vi "PH_PPPA_PowerUnit.ProcState.vi"(0 "i ref in":refnum<vi>, 2 "state timeout":i32=-1, 4 "state":string, 5 "error in (no error)":errorcluster) -> (14 "i ref out":refnum<vi>, 18 "next state":string, 19 "error out":errorcluster)   [LabVIEW 2014, in "PH_PPPA_PowerUnit.lvlib"]
doc: "This VI represents part of the internal state machine of the object. All methods that are needed to implement the required functionality of the state machine will be called from THIS VI. Add your code here."
uses:
  PH_PPPA_PowerUnit.lvlib
  PH_Basics/PH_PowerUnit_BaseClass/PH_PowerUnit_BaseClass.SM States.ctl
  CS_Core/CSSystem/CoreDefs/CoreDefs.error_type.ctl
  CS_Core/CSSystem/CoreLib/CoreLib.lvlib
  CS_Core/BaseSM/BaseSM.lvlib
  PH_Basics/PH_PSDBWriter/PH_PSDBWriter.lvlib
  PH_Devices/PH_Beckhoff_PP_PU/PH_Beckhoff_PP_PU.lvlib
  PH_Basics/PH_PowerUnit_BaseClass/PH_PowerUnit_BaseClass.lvlib
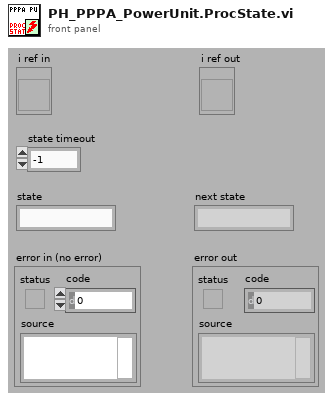
[diagram p1: front panel]
types:
  T1 = typedef "PH_PowerUnit_BaseClass.lvlib/PH_PowerUnit_BaseClass.SM States.ctl" = enum16{".", "Stand by", "Switch PU on", "Configure", "Set Default Voltage", "Set STANDBY", "Set READY", "Wait for Shot Cmd", "Open Dump Rods", "Open Ross Relais", "Close Ross Relais", "Switch PSU on", "Switch PSU off", "Charge", "Switch GD Channel on", "Close Dump Rods", "Rods-TO", "RR-TO", "PSU-TO", "Trigger-TO"}
  T2 = typedef "CoreDefs.error_type.ctl" = enum16{"no error", "can't load process", "can't unload process", "process does not exist", "can't install process", "can't remove process", "unknown function", "time out", "can't execute function", "duplicate queue name", "super not found", "caller queue invalid", "can't ping process", "unknown error", "VISA Error", "VISA timeout", "GPIB timeout", "GPIB error", "communication error", "data type mismatch", "can't read data from OPC server", "can't write data to OPC server", "OET error", "function not implemented", "process already exists", "invalid Shared Variable name", "error writing Shared Variable", "error reading Shared Variable", "invalid client name", "corrupt database", "unknown class", "call not authorized", "parameter out of range", "OET timeout: can't get data to modify", "invalid queue name", "requested operation incompatible with current state", "event undefined", "event disabled", "state undefined", "caller is not a friend", "EventBuilder: bad eventID", "EventBuilder: no DAQ devices", "a thread must not stop itself", "UNUSED ELEMENT4", "DiscArchiver: eventData incomplete", "DiscArchiver: eventData does not belong to run", "DiscArchiver: can't open file", "DiscArchiver: can't write to file", "DiscArchiver: available disc space low", "can't acquire semaphore", "error reading data from database", "notifier object is not existing", "can't register process", "can't unregister process", "illegal event type", "object disabled", "object already exists", "can't change state", "Instrument not found", "no connection to remote node", "invalid reference", "N/A", "UNUSED ELEMENT 1", "element not found", "illegal TCP/IP connection detected", "object does not exist", "invalid access ID", "unknown CS system", "invalid privilige", "unsupported data type", "unsupported server type", "IO server already exists", "Shared Variable already exists"}
  T3 = typedef "PH_PowerUnit_BaseClass.lvlib/PH_PowerUnit_BaseClass.i attribute.ctl" = cluster{"Constructor finished":bool, "PU":cluster{"In use":bool, "Service ID in use":i32, "GUI Ref":refnum<vi>}, "Enabling":cluster{"State":T4, "GUI Ref":refnum<vi>}, "Timing":cluster{"Last Shot":dbl, "Time between Shots [Sec]":dbl, "Waiting Time over?":bool, "Service ID Waiting Time":i32, "GUI Ref":refnum<vi>, "Instance":cluster{"Status":T5, "linked?":bool, "GUI Ref":refnum<vi>}}, "Sequencer":cluster{"SM State":string, "GUI Ref":refnum<vi>, "linked":bool}, "Subscribed Trendmssgs":cluster{"Tagname":string, "Status":T5, "linked?":bool, "Shot Condition":T5, "GUI Ref":refnum<vi>}[], "PP PU":T6, "Default Voltage (V)":dbl, "GUI Refs":T7, "PSDB data":cluster{"Shot Voltage [V]":dbl, "State TO SM":T1, "Write 2 early":bool}, "State TO SM":T1}
  T4 = typedef "PH_SystemInformation.lvlib/PH_SystemInformationEnabling State.ctl" = i32
  T5 = typedef "PH_StatusHandler.lvlib/PH_StatusHandler.Status.ctl" = i16
  T6 = typedef "PH_PP_Common.lvlib/PH_PP_Common.PUs.ctl" = enum16{"no Info", "PA-19mm-1", "PA-19mm-2", "PA-45mm-PILC", "PA-45mm-MAIN", "MA-PU-1", "MA-PU-2", "MA-PU-3", "MA-PU-4", "MA-PU-5", "MA-PU-6", "MA-FR", "MA-PILC", "PA-45mm-DP"}
  T7 = typedef "PH_PowerUnit_BaseClass.lvlib/PH_PowerUnit_BaseClass.GUI Refs.ctl" = cluster{"Delete Inst":refnum<vi>, "State TO SM":refnum<vi>, "State SM":refnum<vi>, "Fire":refnum<vi>}
  T8 = typedef "PH_PPPA_PowerUnit.lvlib/PH_PPPA_PowerUnit.i attribute.ctl" = cluster{"GUI Refs":cluster{"Ignitron":refnum<vi>, "Rossrelais":refnum<vi>, "Set Voltage":refnum<vi>, "PSU":refnum<vi>, "EOC":refnum<vi>, "Trigger":refnum<vi>}, "Ignitron":T9, "PSU":T10, "Dump Ross Relais":T11, "Trigger":cluster{"State Device":T5, "linked?":bool}, "Timing Settings":cluster{"Prdc Fast?":bool, "Default Value Periodic Interval":i32, "Mercury on since":dbl, "Warm up Time Mercury [s]":dbl}, "Set Voltage [V]":dbl, "19er Ignitionbox":string}
  T9 = typedef "PH_PP_Common.lvlib/PH_PP_Common.Ignitron Attributes.ctl" = cluster{"State Device":T5, "linked?":bool}
  T10 = typedef "PH_PP_Common.lvlib/PH_PP_Common.PSU Attributes.ctl" = cluster{"lower limit [V]":dbl, "upper limit [V]":dbl, "Voltage set":bool, "State Device":T5, "linked?":bool}
  T11 = typedef "PH_PP_Common.lvlib/PH_PP_Common.Ross Relais Attributes.ctl" = cluster{"State Device":T5, "linked?":bool}
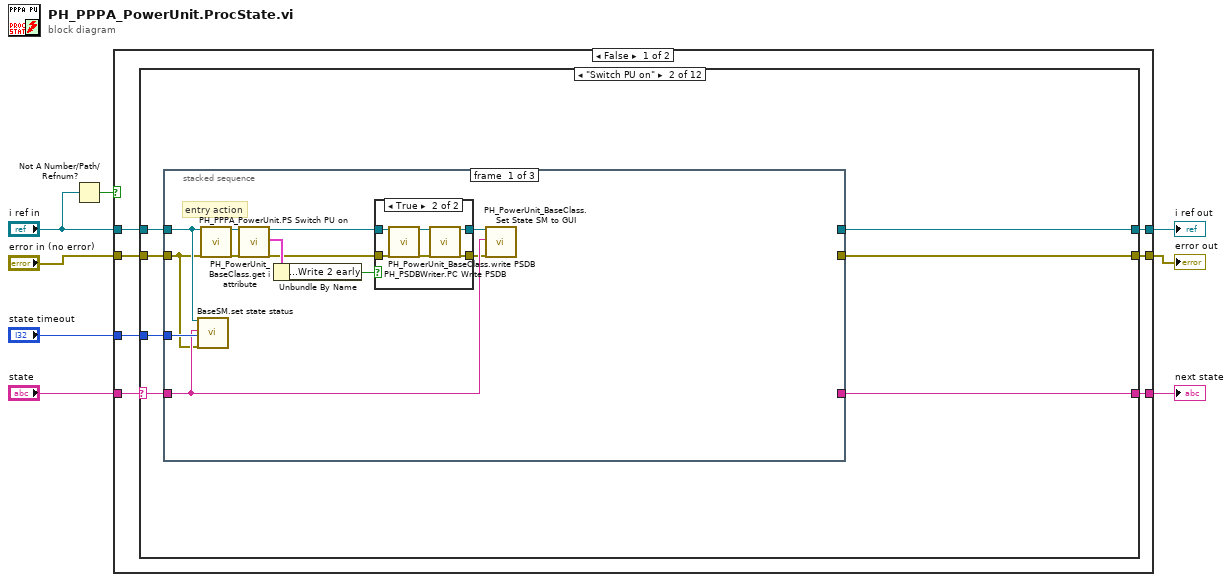
[diagram p0: block diagram]
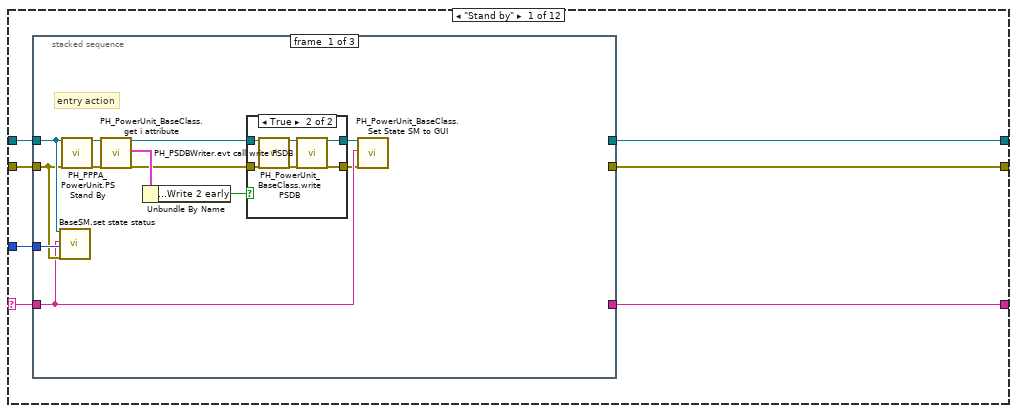
[diagram p2: hidden frame]
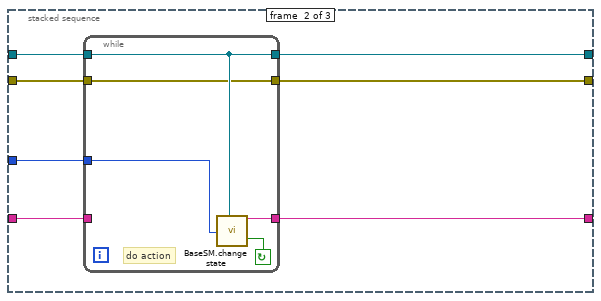
[diagram p4: hidden frame]
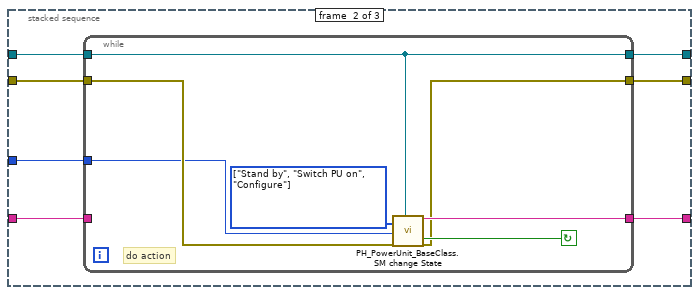
[diagram p7: hidden frame]
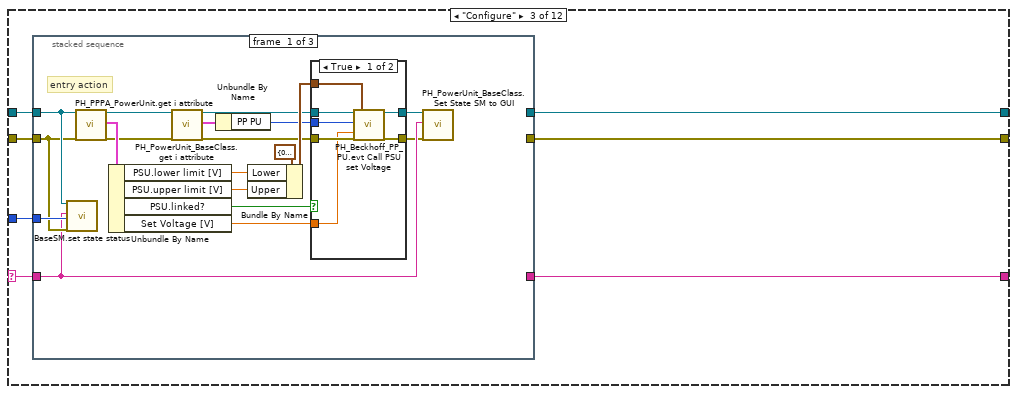
[diagram p9: hidden frame]
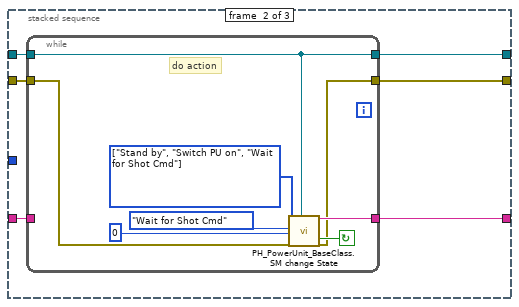
[diagram p11: hidden frame]
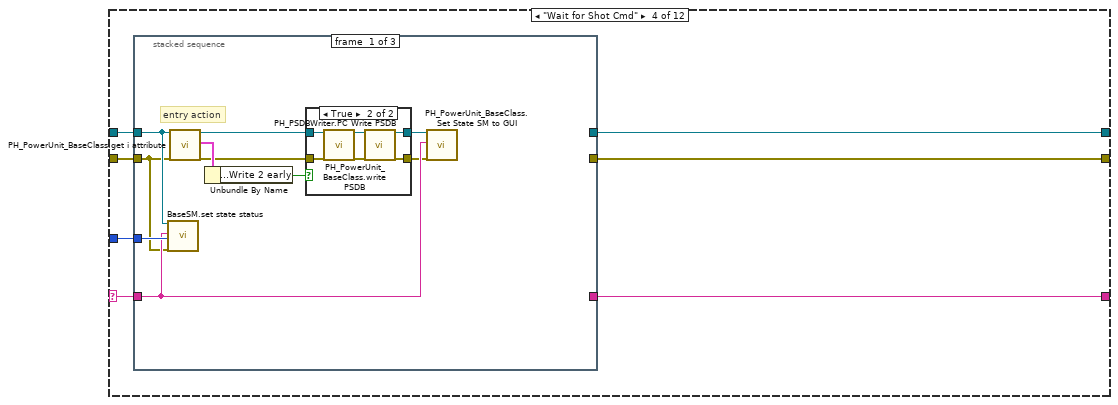
[diagram p13: hidden frame]
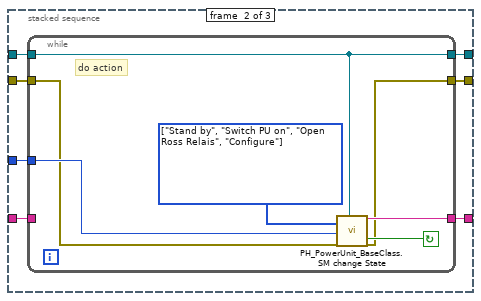
[diagram p15: hidden frame]
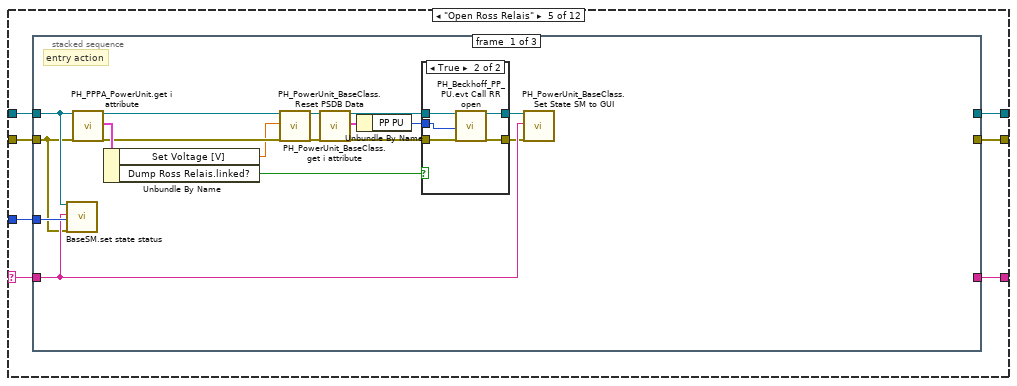
[diagram p17: hidden frame]
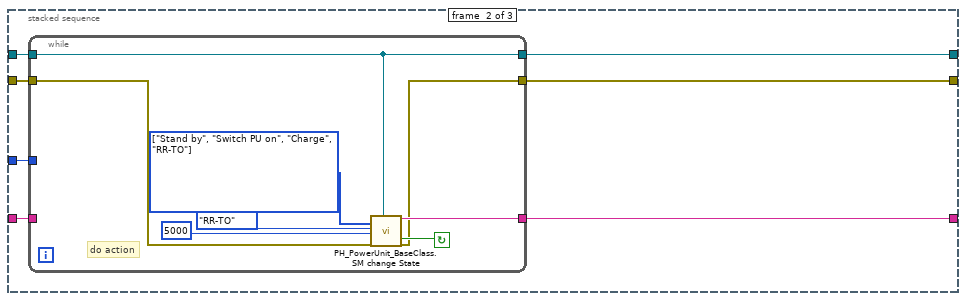
[diagram p19: hidden frame]
diagram:
  n1 = Not A Number/Path/Refnum?(number/path/refnum="i ref in") -> (NaN/Path/Refnum?=w2:bool)
  n2 = case shown="False" w2 {
    tunnel: "i ref in" -> [w15 w435]
    tunnel: [w14 w435] -> w8
    tunnel: "state" -> [w13 w432]
    tunnel: [w12 w432] -> w6
    tunnel: "state timeout" -> [w11 _]
    tunnel: "error in (no error)" -> [w10 _]
    tunnel: [w9 w433] -> w3
    frame False {
      n3 = case shown="\"Switch PU on\"" w13 {
        selector: w13 -> [w22 w61 w102 w151 w190 w236 w298 w323 w350 w377 w404 w426]
        tunnel: w15 -> [w20 w59 w100 w149 w188 w234 w296 w321 w348 w375 w402 w431]
        tunnel: [w19 w58 w99 w148 w187 w233 w295 w320 w347 w374 w401 w430] -> w14
        tunnel: [w21 w60 w101 w150 w189 w235 w297 w322 w349 w376 w403 w425] -> w12
        tunnel: w11 -> [w18 w57 w98 w147 w186 w232 w294 w319 w346 w373 w400 w427]
        tunnel: w10 -> [w17 w56 w97 w146 w185 w231 w293 w318 w345 w372 w399 w429]
        tunnel: [w16 w55 w96 w145 w184 w230 w292 w317 w344 w371 w398 w428] -> w9
        frame "Stand by" {
          n4 = stacked-sequence {
            tunnel: w22 -> [w31 w49 _]
            tunnel: [_ w48 _] -> w21
            tunnel: w20 -> [w33 w46 _]
            tunnel: [_ w45 _] -> w19
            tunnel: w18 -> [w34 w47 _]
            tunnel: w17 -> [w32 w43 _]
            tunnel: [_ w44 _] -> w16
            frame #0 {
              # "entry action"
              n5 = call "BaseSM.set state status.vi"("i ref in"=w33, "stateStatus"=w31, "ms timeout (10000)"=w34, "error in (no error)"=w32) -> ()  [unwired: 13 in, 3 out]
              n6 = call "PH_PPPA_PowerUnit.PS Stand By.vi"("i ref in"=w33, "error in (no error)"=w32) -> ("i ref out"=w29:refnum<vi>, "error out"=w28:errorcluster)  [unwired: 16 in]
              n7 = call "PH_PowerUnit_BaseClass.get i attribute.vi"("i ref in"=w29, "error in (no error)"=w28) -> ("i ref out"=w27:refnum<vi>, "i attribute"=w30:T3, "error out"=w26:errorcluster)  [unwired: 15 in]
              n8 = Unbundle By Name(w30) -> ("PSDB data.Write 2 early"=w25:bool)
              n9 = case shown="True" w25 {
                tunnel: [w36 w38] -> w24
                tunnel: [w35 w37] -> w23
                tunnel: w27 -> [w36 w42]
                tunnel: w26 -> [w35 w41]
                frame False {
                }
                frame True {
                  n10 = call "PH_PowerUnit_BaseClass.write PSDB.vi"("i ref in"=w42, "error IO"=w41) -> ("i ref out"=w39:refnum<vi>, "error out"=w40:errorcluster)  [unwired: 16 in]
                  n11 = call "PH_PSDBWriter.evt call write PSDB.vi"("i ref in"=w39, "error in (no error)"=w40) -> ("i ref out"=w38:refnum<vi>, "error out"=w37:errorcluster)  [unwired: 16 in]
                }
              }
              n12 = call "PH_PowerUnit_BaseClass.Set State SM to GUI.vi"("i ref in"=w24, "State SM"=w31, "error in (no error)"=w23) -> ()  [unwired: 15 in, 2 out]
            }
            frame #1 {
              n13 = while {
                tunnel: w47 -> [w52]
                tunnel: [w54] -> w48
                tunnel: w49 -> [_]
                tunnel: w46 -> [w51]
                tunnel: [w51] -> w45
                tunnel: [w50] -> w44
                tunnel: w43 -> [w50]
                stop <- w53 continue-if-true
                # "do action"
                n14 = call "BaseSM.change state.vi"("wait time [ms]"=w52, "i ref in"=w51) -> ("next state"=w54:string, "continue loop"=w53:bool)  [unwired: 14 in, 2 out]
              }
            }
            frame #2 {
              # "exit action"
            }
          }
        }
        frame "Switch PU on" {
          n15 = stacked-sequence {
            tunnel: w61 -> [w72 w88 _]
            tunnel: [_ w87 _] -> w60
            tunnel: w59 -> [w71 w86 _]
            tunnel: [_ w85 _] -> w58
            tunnel: w57 -> [w73 w82 _]
            tunnel: w56 -> [w70 w83 _]
            tunnel: [_ w84 _] -> w55
            frame #0 {
              # "entry action"
              n16 = call "BaseSM.set state status.vi"("i ref in"=w71, "stateStatus"=w72, "ms timeout (10000)"=w73, "error in (no error)"=w70) -> ()  [unwired: 13 in, 3 out]
              n17 = call "PH_PPPA_PowerUnit.PS Switch PU on.vi"("i ref in"=w71, "error in (no error)"=w70) -> ("i ref out"=w65:refnum<vi>, "error out"=w64:errorcluster)  [unwired: 16 in]
              n18 = call "PH_PowerUnit_BaseClass.get i attribute.vi"("i ref in"=w65, "error in (no error)"=w64) -> ("i ref out"=w68:refnum<vi>, "i attribute"=w69:T3, "error out"=w67:errorcluster)  [unwired: 15 in]
              n19 = Unbundle By Name(w69) -> ("PSDB data.Write 2 early"=w66:bool)
              n20 = case shown="True" w66 {
                tunnel: w68 -> [w75 w77]
                tunnel: w67 -> [w74 w76]
                tunnel: [w75 w79] -> w63
                tunnel: [w74 w78] -> w62
                frame False {
                }
                frame True {
                  n21 = call "PH_PowerUnit_BaseClass.write PSDB.vi"("i ref in"=w77, "error IO"=w76) -> ("i ref out"=w80:refnum<vi>, "error out"=w81:errorcluster)  [unwired: 16 in]
                  n22 = call "PH_PSDBWriter.PC Write PSDB.vi"("i ref in"=w80, "error IO"=w81) -> ("i ref out"=w79:refnum<vi>, "error out"=w78:errorcluster)  [unwired: 16 in]
                }
              }
              n23 = call "PH_PowerUnit_BaseClass.Set State SM to GUI.vi"("i ref in"=w63, "State SM"=w72, "error in (no error)"=w62) -> ()  [unwired: 15 in, 2 out]
            }
            frame #1 {
              n24 = while {
                tunnel: [w95] -> w87
                tunnel: w88 -> [_]
                tunnel: w86 -> [w93]
                tunnel: [w93] -> w85
                tunnel: [w91] -> w84
                tunnel: w83 -> [w92]
                tunnel: w82 -> [w90]
                stop <- w94 continue-if-true
                w89 = T1[] [enum."Stand by", enum."Switch PU on", enum."Configure"] items=[".", "Stand by", "Switch PU on", "Configure", "Set Default Voltage", "Set STANDBY", "Set READY", "Wait for Shot Cmd", "Open Dump Rods", "Open Ross Relais", "Close Ross Relais", "Switch PSU on", "Switch PSU off", "Charge", "Switch GD Channel on", "Close Dump Rods", "Rods-TO", "RR-TO", "PSU-TO", "Trigger-TO"] ("allowed next states")
                # "do action"
                n25 = call "PH_PowerUnit_BaseClass.SM change State.vi"("allowed next states"=w89, "wait time [ms]"=w90, "error in (no error)"=w92, "VI in"=w93) -> ("next state"=w95:string, "continue loop"=w94:bool, "error out"=w91:errorcluster)  [unwired: 13 in]
              }
            }
            frame #2 {
              # "exit action"
            }
          }
        }
        frame "Configure" {
          n26 = stacked-sequence {
            tunnel: w102 -> [w118 w136 _]
            tunnel: [_ w135 _] -> w101
            tunnel: w100 -> [w120 w134 _]
            tunnel: [_ w133 _] -> w99
            tunnel: w98 -> [w121 _ _]
            tunnel: w97 -> [w119 w131 _]
            tunnel: [_ w132 _] -> w96
            frame #0 {
              # "entry action"
              n27 = call "BaseSM.set state status.vi"("i ref in"=w120, "stateStatus"=w118, "ms timeout (10000)"=w121, "error in (no error)"=w119) -> ()  [unwired: 13 in, 3 out]
              n28 = call "PH_PPPA_PowerUnit.get i attribute.vi"("i ref in"=w120, "error in (no error)"=w119) -> ("i ref out"=w106:refnum<vi>, "i attribute"=w117:T8, "error out"=w105:errorcluster)  [unwired: 15 in]
              n29 = Unbundle By Name(w117) -> ("PSU.lower limit [V]"=w112:dbl, "PSU.upper limit [V]"=w111:dbl, "PSU.linked?"=w115:bool, "Set Voltage [V]"=w116:dbl)
              n30 = call "PH_PowerUnit_BaseClass.get i attribute.vi"("i ref in"=w106, "error in (no error)"=w105) -> ("i ref out"=w109:refnum<vi>, "i attribute"=w108:T3, "error out"=w110:errorcluster)  [unwired: 15 in]
              n31 = Unbundle By Name(w108) -> ("PP PU"=w107:T6)
              n32 = Bundle By Name(cluster=cluster{"Lower":dbl, "Upper":dbl} {"Lower"=0.0, "Upper"=0.0} ("Limits [V]"), "Lower"=w112, "Upper"=w111) -> (w113:cluster{"Lower":dbl, "Upper":dbl})
              n33 = case shown="True" w115 {
                tunnel: w109 -> [w128 w130]
                tunnel: w110 -> [w127 w129]
                tunnel: w116 -> [w126 _]
                tunnel: [w125 w130] -> w104
                tunnel: [w124 w129] -> w103
                tunnel: w113 -> [w123 _]
                tunnel: w107 -> [w122 _]
                frame True {
                  n34 = call "PH_Beckhoff_PP_PU.evt Call PSU set Voltage.vi"("i ref in"=w128, "PU"=w122, "Voltage to set [V]"=w126, "error in"=w127, "Limits [V]"=w123) -> ("i ref out"=w125:refnum<vi>, "error out"=w124:errorcluster)  [unwired: 13 in]
                }
                frame False {
                }
              }
              n35 = call "PH_PowerUnit_BaseClass.Set State SM to GUI.vi"("i ref in"=w104, "State SM"=w118, "error in (no error)"=w103) -> ()  [unwired: 15 in, 2 out]
            }
            frame #1 {
              n36 = while {
                tunnel: [w144] -> w135
                tunnel: w136 -> [_]
                tunnel: w134 -> [w142]
                tunnel: [w142] -> w133
                tunnel: [w140] -> w132
                tunnel: w131 -> [w141]
                stop <- w143 continue-if-true
                w137 = T1[] [enum."Stand by", enum."Switch PU on", enum."Wait for Shot Cmd"] items=[".", "Stand by", "Switch PU on", "Configure", "Set Default Voltage", "Set STANDBY", "Set READY", "Wait for Shot Cmd", "Open Dump Rods", "Open Ross Relais", "Close Ross Relais", "Switch PSU on", "Switch PSU off", "Charge", "Switch GD Channel on", "Close Dump Rods", "Rods-TO", "RR-TO", "PSU-TO", "Trigger-TO"] ("allowed next states")
                # "do action"
                n37 = call "PH_PowerUnit_BaseClass.SM change State.vi"("allowed next states"=w137, "default state"=PH_PowerUnit_BaseClass.SM_States."Wait for Shot Cmd", "wait time [ms]"=0 ("wait time"), "error in (no error)"=w141, "VI in"=w142) -> ("next state"=w144:string, "continue loop"=w143:bool, "error out"=w140:errorcluster)  [unwired: 12 in]
              }
            }
            frame #2 {
              # "exit action"
            }
          }
        }
        frame "Wait for Shot Cmd" {
          n38 = stacked-sequence {
            tunnel: w151 -> [w160 w176 _]
            tunnel: [_ w175 _] -> w150
            tunnel: w149 -> [w155 w173 _]
            tunnel: [_ w172 _] -> w148
            tunnel: w147 -> [w161 w174 _]
            tunnel: w146 -> [w154 w170 _]
            tunnel: [_ w171 _] -> w145
            frame #0 {
              # "entry action"
              n39 = call "BaseSM.set state status.vi"("i ref in"=w155, "stateStatus"=w160, "ms timeout (10000)"=w161, "error in (no error)"=w154) -> ()  [unwired: 13 in, 3 out]
              n40 = call "PH_PowerUnit_BaseClass.get i attribute.vi"("i ref in"=w155, "error in (no error)"=w154) -> ("i ref out"=w158:refnum<vi>, "i attribute"=w159:T3, "error out"=w157:errorcluster)  [unwired: 15 in]
              n41 = Unbundle By Name(w159) -> ("PSDB data.Write 2 early"=w156:bool)
              n42 = case shown="True" w156 {
                tunnel: w158 -> [w163 w165]
                tunnel: w157 -> [w162 w164]
                tunnel: [w163 w167] -> w153
                tunnel: [w162 w166] -> w152
                frame False {
                }
                frame True {
                  n43 = call "PH_PowerUnit_BaseClass.write PSDB.vi"("i ref in"=w165, "error IO"=w164) -> ("i ref out"=w168:refnum<vi>, "error out"=w169:errorcluster)  [unwired: 16 in]
                  n44 = call "PH_PSDBWriter.PC Write PSDB.vi"("i ref in"=w168, "error IO"=w169) -> ("i ref out"=w167:refnum<vi>, "error out"=w166:errorcluster)  [unwired: 16 in]
                }
              }
              n45 = call "PH_PowerUnit_BaseClass.Set State SM to GUI.vi"("i ref in"=w153, "State SM"=w160, "error in (no error)"=w152) -> ()  [unwired: 15 in, 2 out]
            }
            frame #1 {
              n46 = while {
                tunnel: w174 -> [w181]
                tunnel: [w183] -> w175
                tunnel: w176 -> [_]
                tunnel: w173 -> [w180]
                tunnel: [w180] -> w172
                tunnel: [w178] -> w171
                tunnel: w170 -> [w179]
                stop <- w182 continue-if-true
                w177 = T1[] [enum."Stand by", enum."Switch PU on", enum."Open Ross Relais", enum."Configure"] items=[".", "Stand by", "Switch PU on", "Configure", "Set Default Voltage", "Set STANDBY", "Set READY", "Wait for Shot Cmd", "Open Dump Rods", "Open Ross Relais", "Close Ross Relais", "Switch PSU on", "Switch PSU off", "Charge", "Switch GD Channel on", "Close Dump Rods", "Rods-TO", "RR-TO", "PSU-TO", "Trigger-TO"] ("allowed next states")
                # "do action"
                n47 = call "PH_PowerUnit_BaseClass.SM change State.vi"("allowed next states"=w177, "wait time [ms]"=w181, "error in (no error)"=w179, "VI in"=w180) -> ("next state"=w183:string, "continue loop"=w182:bool, "error out"=w178:errorcluster)  [unwired: 13 in]
              }
            }
            frame #2 {
              # "exit action"
            }
          }
        }
        frame "Open Ross Relais" {
          n48 = stacked-sequence {
            tunnel: w190 -> [w205 w221 _]
            tunnel: [_ w220 _] -> w189
            tunnel: w188 -> [w199 w218 _]
            tunnel: [_ w217 _] -> w187
            tunnel: w186 -> [w207 w219 _]
            tunnel: w185 -> [w198 w215 _]
            tunnel: [_ w216 _] -> w184
            frame #0 {
              # "entry action"
              n49 = call "BaseSM.set state status.vi"("i ref in"=w199, "stateStatus"=w205, "ms timeout (10000)"=w207, "error in (no error)"=w198) -> ()  [unwired: 13 in, 3 out]
              n50 = call "PH_PPPA_PowerUnit.get i attribute.vi"("i ref in"=w199, "error in (no error)"=w198) -> ("i ref out"=w195:refnum<vi>, "i attribute"=w206:T8, "error out"=w197:errorcluster)  [unwired: 15 in]
              n51 = Unbundle By Name(w206) -> ("Set Voltage [V]"=w193:dbl, "Dump Ross Relais.linked?"=w204:bool)
              n52 = call "PH_PowerUnit_BaseClass.Reset PSDB Data.vi"("VI in"=w195, "PSDB data.Shot Voltage [V]"=w193, "error in (no error)"=w197) -> ("VI out"=w194:refnum<vi>, "error out"=w196:errorcluster)  [unwired: 15 in]
              n53 = call "PH_PowerUnit_BaseClass.get i attribute.vi"("i ref in"=w194, "error in (no error)"=w196) -> ("i ref out"=w202:refnum<vi>, "i attribute"=w201:T3, "error out"=w203:errorcluster)  [unwired: 15 in]
              n54 = Unbundle By Name(w201) -> ("PP PU"=w200:T6)
              n55 = case shown="True" w204 {
                tunnel: w202 -> [w209 w214]
                tunnel: w203 -> [w208 w213]
                tunnel: [w208 w212] -> w191
                tunnel: [w209 w211] -> w192
                tunnel: w200 -> [_ w210]
                frame False {
                }
                frame True {
                  n56 = call "PH_Beckhoff_PP_PU.evt Call RR open.vi"("i ref in"=w214, "PU"=w210, "error in"=w213) -> ("i ref out"=w211:refnum<vi>, "error out"=w212:errorcluster)  [unwired: 15 in]
                }
              }
              n57 = call "PH_PowerUnit_BaseClass.Set State SM to GUI.vi"("i ref in"=w192, "State SM"=w205, "error in (no error)"=w191) -> ()  [unwired: 15 in, 2 out]
            }
            frame #1 {
              n58 = while {
                tunnel: w219 -> [_]
                tunnel: [w229] -> w220
                tunnel: w221 -> [_]
                tunnel: w218 -> [w227]
                tunnel: [w227] -> w217
                tunnel: [w224] -> w216
                tunnel: w215 -> [w225]
                stop <- w228 continue-if-true
                w222 = T1[] [enum."Stand by", enum."Switch PU on", enum."Charge", enum."RR-TO"] items=[".", "Stand by", "Switch PU on", "Configure", "Set Default Voltage", "Set STANDBY", "Set READY", "Wait for Shot Cmd", "Open Dump Rods", "Open Ross Relais", "Close Ross Relais", "Switch PSU on", "Switch PSU off", "Charge", "Switch GD Channel on", "Close Dump Rods", "Rods-TO", "RR-TO", "PSU-TO", "Trigger-TO"] ("allowed next states")
                # "do action"
                n59 = call "PH_PowerUnit_BaseClass.SM change State.vi"("allowed next states"=w222, "default state"=PH_PowerUnit_BaseClass.SM_States."RR-TO", "wait time [ms]"=5000 ("wait time"), "error in (no error)"=w225, "VI in"=w227) -> ("next state"=w229:string, "continue loop"=w228:bool, "error out"=w224:errorcluster)  [unwired: 12 in]
              }
            }
            frame #2 {
              # "exit action"
            }
          }
        }
        frame "Charge" {
          n60 = stacked-sequence {
            tunnel: w236 -> [w244 w283 _]
            tunnel: [_ w282 _] -> w235
            tunnel: w234 -> [w249 w281 _]
            tunnel: [_ w280 _] -> w233
            tunnel: w232 -> [w250 _ _]
            tunnel: w231 -> [w248 w278 _]
            tunnel: [_ w279 _] -> w230
            frame #0 {
              # "entry action"
              n61 = call "BaseSM.set state status.vi"("i ref in"=w249, "stateStatus"=w244, "ms timeout (10000)"=w250, "error in (no error)"=w248) -> ()  [unwired: 13 in, 3 out]
              n62 = call "PH_PPPA_PowerUnit.get i attribute.vi"("i ref in"=w249, "error in (no error)"=w248) -> ("i ref out"=w237:refnum<vi>, "i attribute"=w247:T8, "error out"=w238:errorcluster)  [unwired: 15 in]
              n63 = Unbundle By Name(w247) -> ("PSU.linked?"=w243:bool)
              n64 = call "PH_PowerUnit_BaseClass.get i attribute.vi"("i ref in"=w237, "error in (no error)"=w238) -> ("i ref out"=w241:refnum<vi>, "i attribute"=w240:T3, "error out"=w242:errorcluster)  [unwired: 15 in]
              n65 = Unbundle By Name(w240) -> ("PP PU"=w239:T6)
              n66 = case shown="True" w243 {
                tunnel: w241 -> [w261 w277]
                tunnel: w242 -> [w260 w276]
                tunnel: [w252 w276] -> w245
                tunnel: [w251 w277] -> w246
                tunnel: w239 -> [w259 _]
                frame True {
                  n67 = flat-sequence {
                    tunnel: w261 -> [w266]
                    tunnel: w260 -> [w264]
                    tunnel: w259 -> [w262]
                    tunnel: [w265] -> w258
                    tunnel: [w263] -> w257
                    tunnel: [w262] -> w256
                    tunnel: w258 -> [w270]
                    tunnel: w257 -> [w269]
                    tunnel: w256 -> [w268]
                    tunnel: [w270] -> w255
                    tunnel: [w269] -> w254
                    tunnel: [w268] -> w253
                    tunnel: [w272] -> w252
                    tunnel: [w274] -> w251
                    tunnel: w255 -> [w275]
                    tunnel: w254 -> [w273]
                    tunnel: w253 -> [w271]
                    frame #0 {
                      n68 = call "PH_Beckhoff_PP_PU.evt Call PSU Inhibit off.vi"("i ref in"=w266, "PU"=w262, "error in"=w264) -> ("i ref out"=w265:refnum<vi>, "error out"=w263:errorcluster)  [unwired: 15 in]
                    }
                    frame #1 {
                      n69 = Wait (ms)(milliseconds to wait=u32 1500) -> ()  [unwired: 1 out]
                    }
                    frame #2 {
                      n70 = call "PH_Beckhoff_PP_PU.evt Call PSU HV on.vi"("i ref in"=w275, "PU"=w271, "error in"=w273) -> ("i ref out"=w274:refnum<vi>, "error out"=w272:errorcluster)  [unwired: 15 in]
                    }
                  }
                }
                frame False {
                }
              }
              n71 = call "PH_PowerUnit_BaseClass.Set State SM to GUI.vi"("i ref in"=w246, "State SM"=w244, "error in (no error)"=w245) -> ()  [unwired: 15 in, 2 out]
            }
            frame #1 {
              n72 = while {
                tunnel: [w291] -> w282
                tunnel: w283 -> [_]
                tunnel: w281 -> [w289]
                tunnel: [w289] -> w280
                tunnel: [w286] -> w279
                tunnel: w278 -> [w287]
                stop <- w290 continue-if-true
                w284 = T1[] [enum."Stand by", enum."Switch PU on", enum."Switch GD Channel on", enum."PSU-TO"] items=[".", "Stand by", "Switch PU on", "Configure", "Set Default Voltage", "Set STANDBY", "Set READY", "Wait for Shot Cmd", "Open Dump Rods", "Open Ross Relais", "Close Ross Relais", "Switch PSU on", "Switch PSU off", "Charge", "Switch GD Channel on", "Close Dump Rods", "Rods-TO", "RR-TO", "PSU-TO", "Trigger-TO"] ("allowed next states")
                # "do action"
                n73 = call "PH_PowerUnit_BaseClass.SM change State.vi"("allowed next states"=w284, "default state"=PH_PowerUnit_BaseClass.SM_States."PSU-TO", "wait time [ms]"=45000 ("wait time"), "error in (no error)"=w287, "VI in"=w289) -> ("next state"=w291:string, "continue loop"=w290:bool, "error out"=w286:errorcluster)  [unwired: 12 in]
              }
            }
            frame #2 {
              # "exit action"
            }
          }
        }
        frame "Switch GD Channel on" {
          n74 = stacked-sequence {
            tunnel: w298 -> [w301 w308 _]
            tunnel: [_ w307 _] -> w297
            tunnel: w296 -> [w300 w306 _]
            tunnel: [_ w305 _] -> w295
            tunnel: w294 -> [w302 _ _]
            tunnel: w293 -> [w299 w303 _]
            tunnel: [_ w304 _] -> w292
            frame #0 {
              # "entry action"
              n75 = call "BaseSM.set state status.vi"("i ref in"=w300, "stateStatus"=w301, "ms timeout (10000)"=w302, "error in (no error)"=w299) -> ()  [unwired: 13 in, 3 out]
              n76 = call "PH_PowerUnit_BaseClass.Set State SM to GUI.vi"("i ref in"=w300, "State SM"=w301, "error in (no error)"=w299) -> ()  [unwired: 15 in, 2 out]
            }
            frame #1 {
              n77 = while {
                tunnel: [w316] -> w307
                tunnel: w308 -> [_]
                tunnel: w306 -> [w312]
                tunnel: [w312] -> w305
                tunnel: [w314] -> w304
                tunnel: w303 -> [w311]
                stop <- w315 continue-if-true
                w309 = T1[] [enum."Stand by", enum."Switch PU on", enum."Close Ross Relais", enum."Trigger-TO"] items=[".", "Stand by", "Switch PU on", "Configure", "Set Default Voltage", "Set STANDBY", "Set READY", "Wait for Shot Cmd", "Open Dump Rods", "Open Ross Relais", "Close Ross Relais", "Switch PSU on", "Switch PSU off", "Charge", "Switch GD Channel on", "Close Dump Rods", "Rods-TO", "RR-TO", "PSU-TO", "Trigger-TO"] ("allowed next states")
                # "do action"
                n78 = call "PH_PowerUnit_BaseClass.SM change State.vi"("allowed next states"=w309, "default state"=PH_PowerUnit_BaseClass.SM_States."Trigger-TO", "wait time [ms]"=60000, "error in (no error)"=w311, "VI in"=w312) -> ("next state"=w316:string, "continue loop"=w315:bool, "error out"=w314:errorcluster)  [unwired: 12 in]
              }
            }
            frame #2 {
              # "exit action"
            }
          }
        }
        frame "Close Ross Relais" {
          n79 = stacked-sequence {
            tunnel: w323 -> [w328 w335 _]
            tunnel: [_ w334 _] -> w322
            tunnel: w321 -> [w327 w333 _]
            tunnel: [_ w332 _] -> w320
            tunnel: w319 -> [w329 _ _]
            tunnel: w318 -> [w326 w330 _]
            tunnel: [_ w331 _] -> w317
            frame #0 {
              # "entry action"
              n80 = call "BaseSM.set state status.vi"("i ref in"=w327, "stateStatus"=w328, "ms timeout (10000)"=w329, "error in (no error)"=w326) -> ()  [unwired: 13 in, 3 out]
              n81 = call "PH_PPPA_PowerUnit.PS Close RR.vi"("i ref in"=w327, "error in (no error)"=w326) -> ("i ref out"=w325:refnum<vi>, "error out"=w324:errorcluster)  [unwired: 16 in]
              n82 = call "PH_PowerUnit_BaseClass.Set State SM to GUI.vi"("i ref in"=w325, "State SM"=w328, "error in (no error)"=w324) -> ()  [unwired: 15 in, 2 out]
            }
            frame #1 {
              n83 = while {
                tunnel: [w343] -> w334
                tunnel: w335 -> [_]
                tunnel: w333 -> [w341]
                tunnel: [w341] -> w332
                tunnel: [w339] -> w331
                tunnel: w330 -> [w340]
                stop <- w342 continue-if-true
                w336 = T1[] [enum."Stand by", enum."Switch PU on", enum."Wait for Shot Cmd", enum."RR-TO"] items=[".", "Stand by", "Switch PU on", "Configure", "Set Default Voltage", "Set STANDBY", "Set READY", "Wait for Shot Cmd", "Open Dump Rods", "Open Ross Relais", "Close Ross Relais", "Switch PSU on", "Switch PSU off", "Charge", "Switch GD Channel on", "Close Dump Rods", "Rods-TO", "RR-TO", "PSU-TO", "Trigger-TO"] ("allowed next states")
                # "do action"
                n84 = call "PH_PowerUnit_BaseClass.SM change State.vi"("allowed next states"=w336, "default state"=PH_PowerUnit_BaseClass.SM_States."RR-TO", "wait time [ms]"=10000 ("wait time"), "error in (no error)"=w340, "VI in"=w341) -> ("next state"=w343:string, "continue loop"=w342:bool, "error out"=w339:errorcluster)  [unwired: 12 in]
              }
            }
            frame #2 {
              # "exit action"
            }
          }
        }
        frame "RR-TO" {
          n85 = stacked-sequence {
            tunnel: w350 -> [w353 w362 _]
            tunnel: [_ w361 _] -> w349
            tunnel: w348 -> [w352 w360 _]
            tunnel: [_ w359 _] -> w347
            tunnel: w346 -> [w356 _ _]
            tunnel: w345 -> [w351 w357 _]
            tunnel: [_ w358 _] -> w344
            frame #0 {
              # "entry action"
              n86 = call "BaseSM.set state status.vi"("i ref in"=w352, "stateStatus"=w353, "ms timeout (10000)"=w356, "error in (no error)"=w351) -> ()  [unwired: 13 in, 3 out]
              n87 = call "PH_PowerUnit_BaseClass.handle TO.vi"("VI in"=w352, "String"=w353, "error in (no error)"=w351) -> ("VI out"=w355:refnum<vi>, "error out"=w354:errorcluster)  [unwired: 15 in]
              n88 = call "PH_PowerUnit_BaseClass.Set State SM to GUI.vi"("i ref in"=w355, "State SM"=w353, "error in (no error)"=w354) -> ()  [unwired: 15 in, 2 out]
            }
            frame #1 {
              n89 = while {
                tunnel: [w370] -> w361
                tunnel: w362 -> [_]
                tunnel: w360 -> [w368]
                tunnel: [w368] -> w359
                tunnel: [w366] -> w358
                tunnel: w357 -> [w367]
                stop <- w369 continue-if-true
                w363 = T1[] [enum."Stand by", enum."Switch PU on"] items=[".", "Stand by", "Switch PU on", "Configure", "Set Default Voltage", "Set STANDBY", "Set READY", "Wait for Shot Cmd", "Open Dump Rods", "Open Ross Relais", "Close Ross Relais", "Switch PSU on", "Switch PSU off", "Charge", "Switch GD Channel on", "Close Dump Rods", "Rods-TO", "RR-TO", "PSU-TO", "Trigger-TO"] ("allowed next states")
                # "do action"
                n90 = call "PH_PowerUnit_BaseClass.SM change State.vi"("allowed next states"=w363, "default state"=PH_PowerUnit_BaseClass.SM_States."Switch PU on", "wait time [ms]"=0 ("wait time"), "error in (no error)"=w367, "VI in"=w368) -> ("next state"=w370:string, "continue loop"=w369:bool, "error out"=w366:errorcluster)  [unwired: 12 in]
              }
            }
            frame #2 {
              # "exit action"
            }
          }
        }
        frame "PSU-TO" {
          n91 = stacked-sequence {
            tunnel: w377 -> [w382 w389 _]
            tunnel: [_ w388 _] -> w376
            tunnel: w375 -> [w379 w387 _]
            tunnel: [_ w386 _] -> w374
            tunnel: w373 -> [w383 _ _]
            tunnel: w372 -> [w378 w384 _]
            tunnel: [_ w385 _] -> w371
            frame #0 {
              # "entry action"
              n92 = call "BaseSM.set state status.vi"("i ref in"=w379, "stateStatus"=w382, "ms timeout (10000)"=w383, "error in (no error)"=w378) -> ()  [unwired: 13 in, 3 out]
              n93 = call "PH_PowerUnit_BaseClass.handle TO.vi"("VI in"=w379, "String"=w382, "error in (no error)"=w378) -> ("VI out"=w381:refnum<vi>, "error out"=w380:errorcluster)  [unwired: 15 in]
              n94 = call "PH_PowerUnit_BaseClass.Set State SM to GUI.vi"("i ref in"=w381, "State SM"=w382, "error in (no error)"=w380) -> ()  [unwired: 15 in, 2 out]
            }
            frame #1 {
              n95 = while {
                tunnel: [w397] -> w388
                tunnel: w389 -> [_]
                tunnel: w387 -> [w395]
                tunnel: [w395] -> w386
                tunnel: [w393] -> w385
                tunnel: w384 -> [w394]
                stop <- w396 continue-if-true
                w391 = T1[] [enum."Stand by", enum."Switch PU on"] items=[".", "Stand by", "Switch PU on", "Configure", "Set Default Voltage", "Set STANDBY", "Set READY", "Wait for Shot Cmd", "Open Dump Rods", "Open Ross Relais", "Close Ross Relais", "Switch PSU on", "Switch PSU off", "Charge", "Switch GD Channel on", "Close Dump Rods", "Rods-TO", "RR-TO", "PSU-TO", "Trigger-TO"] ("allowed next states")
                # "do action"
                n96 = call "PH_PowerUnit_BaseClass.SM change State.vi"("allowed next states"=w391, "default state"=PH_PowerUnit_BaseClass.SM_States."Switch PU on", "wait time [ms]"=0 ("wait time"), "error in (no error)"=w394, "VI in"=w395) -> ("next state"=w397:string, "continue loop"=w396:bool, "error out"=w393:errorcluster)  [unwired: 12 in]
              }
            }
            frame #2 {
              # "exit action"
            }
          }
        }
        frame "Trigger-TO" {
          n97 = stacked-sequence {
            tunnel: w404 -> [w407 w416 _]
            tunnel: [_ w415 _] -> w403
            tunnel: w402 -> [w406 w414 _]
            tunnel: [_ w413 _] -> w401
            tunnel: w400 -> [w410 _ _]
            tunnel: w399 -> [w405 w411 _]
            tunnel: [_ w412 _] -> w398
            frame #0 {
              # "entry action"
              n98 = call "BaseSM.set state status.vi"("i ref in"=w406, "stateStatus"=w407, "ms timeout (10000)"=w410, "error in (no error)"=w405) -> ()  [unwired: 13 in, 3 out]
              n99 = call "PH_PowerUnit_BaseClass.handle TO.vi"("VI in"=w406, "String"=w407, "error in (no error)"=w405) -> ("VI out"=w409:refnum<vi>, "error out"=w408:errorcluster)  [unwired: 15 in]
              n100 = call "PH_PowerUnit_BaseClass.Set State SM to GUI.vi"("i ref in"=w409, "State SM"=w407, "error in (no error)"=w408) -> ()  [unwired: 15 in, 2 out]
            }
            frame #1 {
              n101 = while {
                tunnel: [w424] -> w415
                tunnel: w416 -> [_]
                tunnel: w414 -> [w418]
                tunnel: [w418] -> w413
                tunnel: [w423] -> w412
                tunnel: w411 -> [w421]
                stop <- w417 continue-if-true
                w419 = T1[] [enum."Stand by", enum."Switch PU on"] items=[".", "Stand by", "Switch PU on", "Configure", "Set Default Voltage", "Set STANDBY", "Set READY", "Wait for Shot Cmd", "Open Dump Rods", "Open Ross Relais", "Close Ross Relais", "Switch PSU on", "Switch PSU off", "Charge", "Switch GD Channel on", "Close Dump Rods", "Rods-TO", "RR-TO", "PSU-TO", "Trigger-TO"] ("SM States")
                # "do action"
                n102 = call "PH_PowerUnit_BaseClass.SM change State.vi"("allowed next states"=w419, "default state"=PH_PowerUnit_BaseClass.SM_States."Switch PU on" ("SM State"), "wait time [ms]"=0 ("wait time"), "error in (no error)"=w421, "VI in"=w418) -> ("next state"=w424:string, "continue loop"=w417:bool, "error out"=w423:errorcluster)  [unwired: 12 in]
              }
            }
            frame #2 {
              # "exit action"
            }
          }
        }
        frame Default {
          n103 = call "BaseSM.ProcState.vi"("i ref in"=w431, "state timeout [ms]"=w427, "state"=w426, "error in (no error)"=w429) -> ("i ref out"=w430:refnum<vi>, "next state"=w425:string, "error out"=w428:errorcluster)  [unwired: 13 in]
        }
      }
    }
    frame True {
      n104 = call "CoreLib.my to LV error.vi"("ErrorTypes"=CoreDefs.error_type."invalid reference") -> ("myErrorCluster"=w433:errorcluster)  [unwired: 17 in, 1 out]
    }
  }
  "i ref out" <- w8
  "next state" <- w6
  "error out" <- w3
